vi "Table.vi"(1 "Table In":string[][](table), 3 "String To Append":string) -> (0 "Table Out":string[][](table))   [LabVIEW 2011]
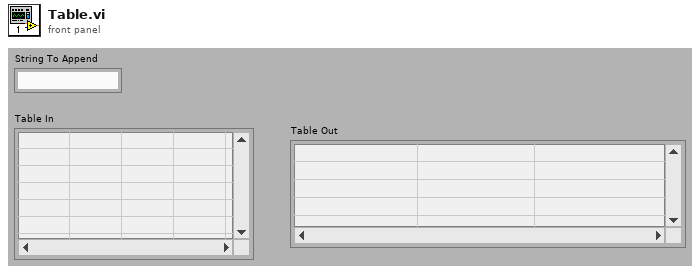
[diagram p1: front panel]
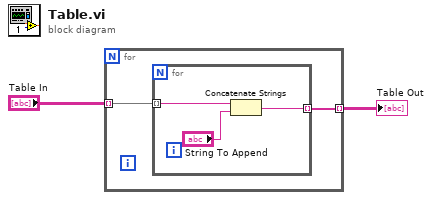
[diagram p0: block diagram]
diagram:
  n1 = for {
    tunnel: "Table In" -> [w4] mode=indexing
    tunnel: [w3] -> w1 mode=indexing
    n2 = for {
      tunnel: w4 -> [w7] mode=indexing
      tunnel: [w5] -> w3 mode=indexing
      n3 = Concatenate Strings(w7, "String To Append") -> (w5:string)
    }
  }
  "Table Out" <- w1
